vi "ZMC Get String Type.vi"(0 "handle":u32, 1 "type2":u32, 5 "sname":string, 7 "filenum":u16, 9 "type":u16, 11 "error in (no error)":errorcluster caption="错误输入（无错误）", 12 "pvalue":dbl) -> (3 "type2 out":u32, 4 "handle out":u32, 6 "function return":i32, 10 "type out":u16, 14 "pvalue out":dbl, 15 "error out":errorcluster caption="错误输出")   [LabVIEW 2015, in "zauxdll.lvlib"]
doc: "int32 __stdcall ZMC_GetStringType(ZMC_HANDLE handle, const char *sname, uint16 filenum, uint16* type, uint32* type2, double *pvalue);"
uses:
  zauxdll.lvlib
  zmotion.dll
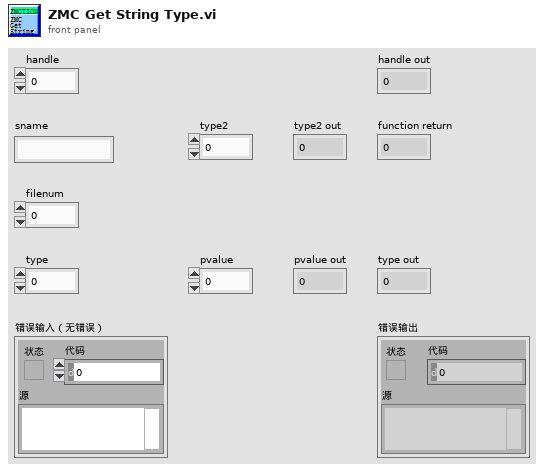
[diagram p1: front panel]
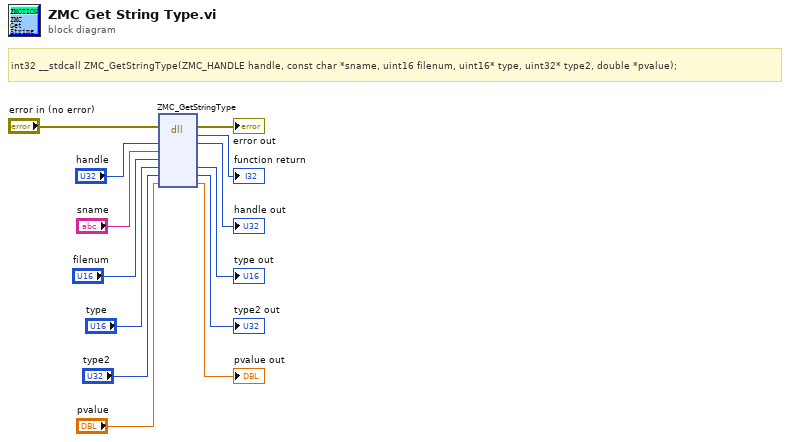
[diagram p0: block diagram]
diagram:
  # "int32 __stdcall ZMC_GetStringType(ZMC_HANDLE handle, const char *sname, uint16 filenum, uint16* type, uint32* type2, double *pvalue);"
  n1 = dll-call lib="C:/Users/VIC/Desktop/GOGORO_SA/system/LLB/zmotion/zaux/zmotion.*" fn="ZMC_GetStringType"(error in="error in (no error)", "handle"="handle", "sname"="sname", "filenum"="filenum", "type"="type", "type2"="type2", "pvalue"="pvalue") -> (error out=→"error out":errorcluster, →"function return":i32, "handle"=→"handle out":u32, "type"=→"type out":u16, "type2"=→"type2 out":u32, "pvalue"=→"pvalue out":dbl)  [unwired: 4 in, 1 out]
